vi "DHE_DRV_load_file.vi"(0 "fd":i32, 5 "dest":i16, 7 "filename":string, 11 "error in (no error)":errorcluster) -> (4 "fd out":i32, 8 "return value":i32, 15 "error out":errorcluster)   [LabVIEW 2016]
doc: "This VI closes the I/O interface with the instrument."
uses:
  c/lib/libarcDHE.so
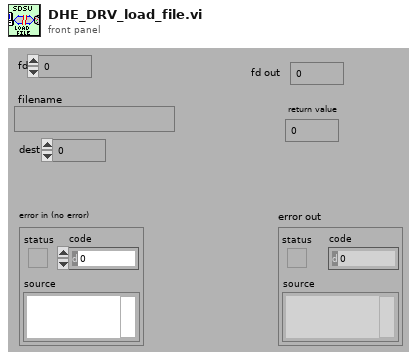
[diagram p1: front panel]
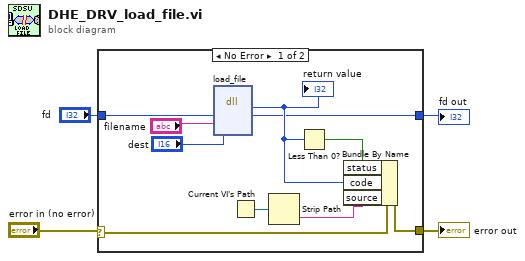
[diagram p0: block diagram]
diagram:
  n1 = case shown="No Error" "error in (no error)" {
    selector: "error in (no error)" -> [w5 w15]
    tunnel: "fd" -> [w14 w16]
    tunnel: [w9 w15] -> w3
    tunnel: [w6 w16] -> w2
    frame No Error {
      n2 = dll-call lib="home/simager/panview/PAN/Modules/SDSU/private/c/lib/libarcDHE.so" fn="load_file"("fd"=w14, "filename"="filename", "dest"="dest") -> (w12:i32, "fd"=w6:i32)  [unwired: 5 in, 2 out]
      "return value" <- w12
      n3 = Current VI's Path() -> (path=w11:path)
      n4 = Strip Path(path=w11) -> (name=w10:string)  [unwired: 1 out]
      n5 = Less Than 0?(x=w12) -> (x < 0?=w13:bool)
      n6 = Bundle By Name(cluster=w5, "status"=w13, "code"=w12, "source"=w10) -> (w9:errorcluster)
    }
    frame Error {
    }
  }
  "error out" <- w3
  "fd out" <- w2
